vi "openref.vi"   [LabVIEW 2014]
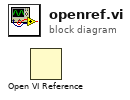
[diagram p0: block diagram]
diagram:
  n1 = Open VI Reference() -> ()  [unwired: 6 in, 2 out]
